vi "DAQ Engineer.vi"(0 "DAQ Name":string="USB-6343", 1 "DAQ Engr Action":T3, 5 "Channel":T2, 7 "Trigger":T1, 9 "Value":dbl, 11 "error in (no error)":errorcluster) -> (4 "device":tag, 14 "Connected":bool, 15 "error out":errorcluster)   [LabVIEW 2015]
uses:
  DAQ Engineer.ctl
  NI DAQs/NI-DAQ6343/Digital Channels.ctl
  NI DAQs/NI-DAQ6343/PFI Channels.ctl
  <vilib>/DAQmx/write.llb/DAQmx Write (Digital Wfm 1Chan NSamp).vi
  <vilib>/DAQmx/write.llb/DAQmx Write (Digital U32 1Chan 1Samp).vi
  <vilib>/Waveform/DWDTOps.llb/DWDT Boolean Array to Digital.vi
  <vilib>/DAQmx/create/channels.llb/DAQmx Create Channel (DO-Digital Output).vi
  <vilib>/DAQmx/configure/timing.llb/DAQmx Timing (Sample Clock).vi
  <vilib>/DAQmx/configure/trigger.llb/DAQmx Start Trigger (Digital Edge).vi
  <vilib>/Waveform/DWDTOps.llb/DWDT Uncompress Digital.vi
  <vilib>/DAQmx/miscellaneous.llb/DAQmx Fill In Error Info.vi
  <vilib>/DAQmx/create/channels.llb/DAQmx Create Channel (DI-Digital Input).vi
panel:
  out "Digital Waveform Graph":digitalwaveform(graph)
  out "ch":string
  out "trigger":string
  # "need three pulses for\nthe instrument to register"
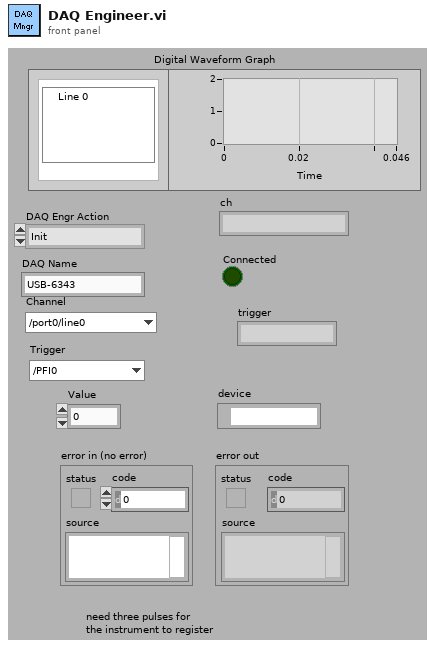
[diagram p1: front panel]
types:
  T1 = typedef "PFI Channels.ctl" = enum16{"/PFI0", "/PFI1", "/PFI2", "/PFI3", "/PFI4", "/PFI5", "/PFI6", "/PFI7", "/PFI8", "/PFI9", "/PFI10", "/PFI11", "/PFI12", "/PFI13", "/PFI14", "/PFI15"}
  T2 = typedef "Digital Channels.ctl" = enum16{"/port0/line0", "/port0/line1", "/port0/line2", "/port0/line3", "/port0/line4", "/port0/line5", "/port0/line6", "/port0/line7", "/port0/line8", "/port0/line9", "/port0/line10", "/port0/line11", "/port0/line12", "/port0/line13", "/port0/line14", "/port0/line15", "/port0/line16", "/port0/line17", "/port0/line18", "/port0/line19", "/port0/line20", "/port0/line21", "/port0/line22", "/port0/line23", "/port0/line24", "/port0/line25", "/port0/line26", "/port0/line27", "/port0/line28", "/port0/line29", "/port0/line30", "/port0/line31"}
  T3 = typedef "DAQ Engineer.ctl" = enum16{"Init", "All Digital Out", "All Digital Input", "DigitalOutOnTrigger", "Close"}
  T4 = cluster{"negative limit switch":bool, "positive limit switch":bool, "home switch":bool, "position marker":bool, "device enable":bool, "quick stop":bool, "general purpose J":bool, "general purpose I":bool, "general purpose H":bool, "general purpose G":bool, "general purpose F":bool, "general purpose E":bool, "general purpose D":bool, "general purpose C":bool, "general purpose B":bool, "general purpose A":bool}
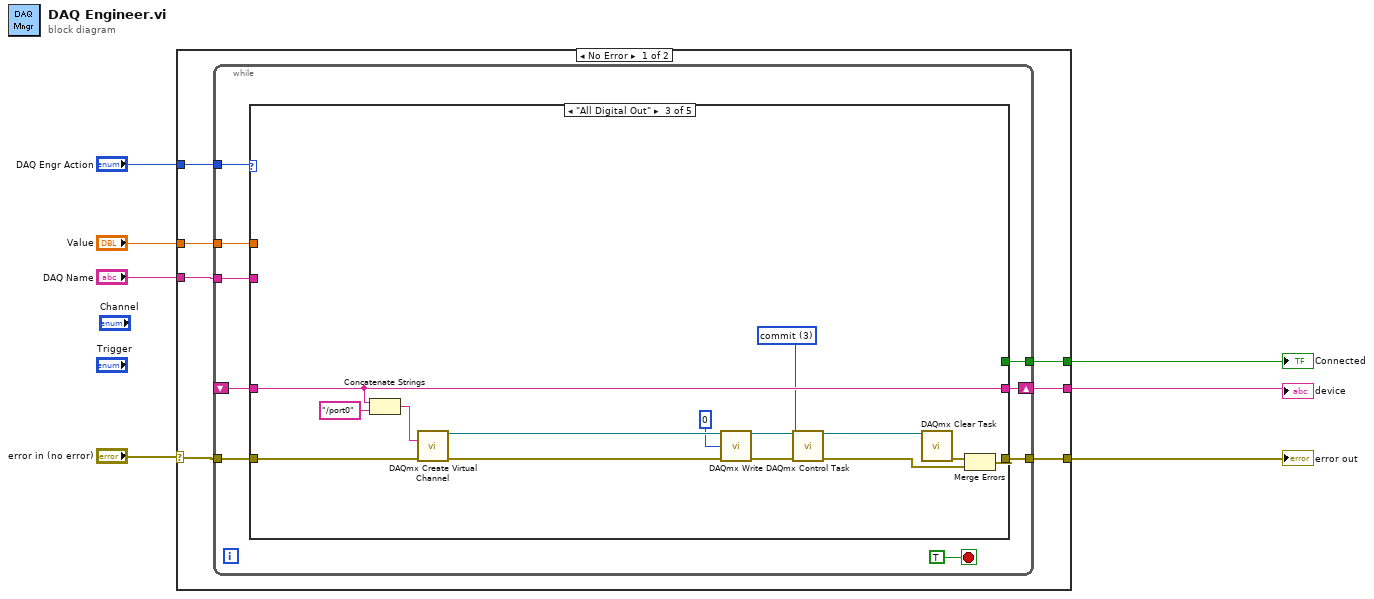
[diagram p0: block diagram]
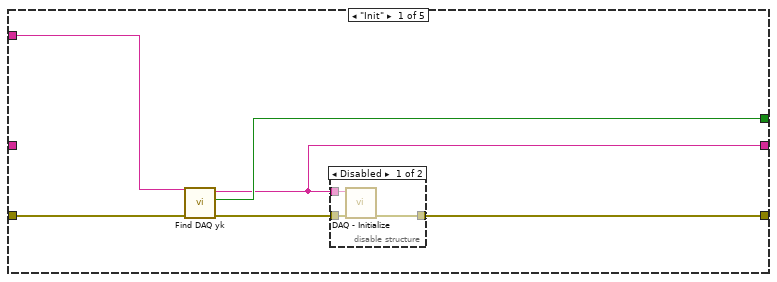
[diagram p2: hidden frame]
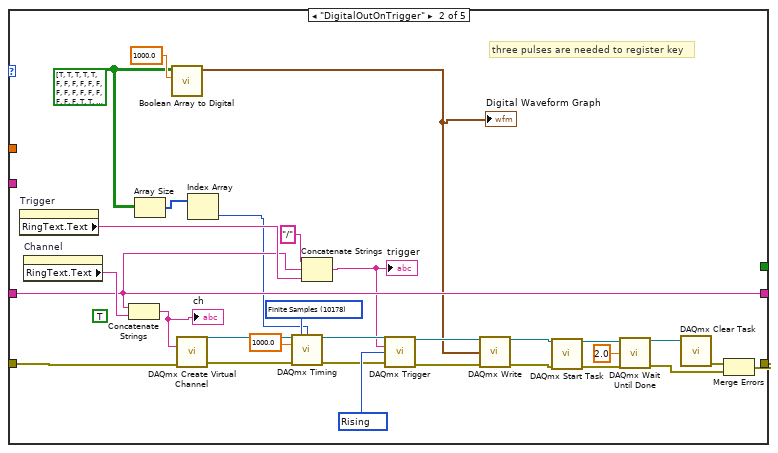
[diagram p4: hidden frame]
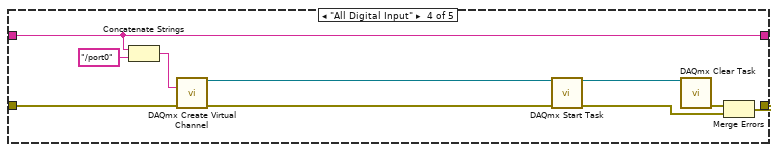
[diagram p5: hidden frame]
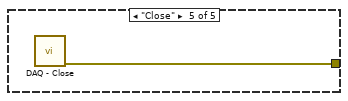
[diagram p6: hidden frame]
diagram:
  n1 = case shown="No Error" "error in (no error)" {
    selector: "error in (no error)" -> [w14 w88]
    tunnel: [w12 w88] -> w6
    tunnel: "DAQ Name" -> [w13 _]
    tunnel: "DAQ Engr Action" -> [w11 _]
    tunnel: [w10 _] -> w3
    tunnel: [w9 _] -> w2
    tunnel: "Value" -> [w8 _]
    frame No Error {
      n2 = while {
        tunnel: w14 -> [w21]
        tunnel: w13 -> [w20]
        tunnel: [w19] -> w12
        tunnel: w11 -> [w22]
        tunnel: [w18] -> w10
        tunnel: w8 -> [w16]
        shift-right: [w17] -> w9
        shift-left: _ -> [w15]
        stop <- TRUE stop-if-true
        n3 = case shown="\"All Digital Out\"" w22 {
          tunnel: w21 -> [w28 w40 w71 w83 _]
          tunnel: w20 -> [w27 _ _ _ _]
          tunnel: [w26 w51 w74 w84 w87] -> w19
          tunnel: [w25 _ _ _ _] -> w18
          tunnel: [w24 w52 w75 w85 _] -> w17
          tunnel: w16 -> [_ _ _ _ _]
          tunnel: w15 -> [_ w52 w75 w85 _]
          frame "Init" {
            n4 = call "Find DAQ yk.vi"("error in"=w28, "DAQ Name"=w27) -> ("error out"=w29:errorcluster, "Device Found"=w25:bool, "device"=w24:tag)  [unwired: 5 in, 2 out]
            n5 = disable-structure shown="Disabled" {
              disable-tunnel: w29 -> [w32 _]
              disable-tunnel: [w31 _] -> w26
              disable-tunnel: w24 -> [w30 _]
              frame Disabled {
                n6 = call "DAQ - Initialize.vi"("error in (no error)"=w32, "DAQ"=w30) -> ("error out"=w31:errorcluster)  [unwired: 9 in]
              }
              frame Enabled {
              }
            }
          }
          frame "DigitalOutOnTrigger" {
            w34 = bool[][] [[TRUE], [TRUE], [TRUE], [TRUE], [TRUE], [FALSE], [FALSE], [FALSE], [FALSE], [FALSE], [FALSE], [FALSE], [FALSE], [FALSE], [FALSE], [FALSE], [FALSE], [FALSE], [FALSE], [FALSE], [TRUE], [TRUE], [TRUE], [TRUE], [TRUE], [FALSE], [FALSE], [FALSE], [FALSE], [FALSE], [FALSE], [FALSE], [FALSE], [FALSE], [FALSE], [FALSE], [FALSE], [FALSE], [FALSE], [FALSE], [TRUE], [TRUE], [TRUE], [TRUE], [TRUE], [FALSE]] ("transposed array")
            w58 = 10178 items=["Finite Samples"=10178, "Continuous Samples"=10123, "Hardware Timed Single Point"=12522] ("sample mode")
            w60 = 10280 items=["Rising"=10280, "Falling"=10171] ("edge")
            (unwired) TRUE ("auto cleanup")
            # "three pulses are needed to register key"
            n7 = property on="Trigger" class="Enum (strict)"() -> ("RingText.Text"=w61:string)  [unwired: 2 in, 2 out]
            n8 = property on="Channel" class="Enum (strict)"() -> ("RingText.Text"=w62:string)  [unwired: 2 in, 2 out]
            n9 = Concatenate Strings(w52, w62) -> (w39:string)
            "ch" <- w39
            n10 = Array Size(array=w34) -> (size(s)=w38:i32[])
            n11 = call-poly <vilib>:"Boolean Array to Digital.vi"("sample rate"=1000.0, "boolean array"=w34) -> ("digital waveform"=w35:digitalwaveform)  [unwired: 8 in, 1 out]
            "Digital Waveform Graph" <- w35
            n12 = call-poly <vilib>:"DAQmx Create Virtual Channel.vi"("lines"=w39, "error in"=w40) -> ("task out"=w55:refnum<k21>, "error out"=w56:errorcluster)  [unwired: 12 in]
            n13 = Index Array(array=w38) -> (element=w37:i32)  [unwired: 1 in]
            n14 = call-poly <vilib>:"DAQmx Timing.vi"("task/channels in"=w55, "sample mode"=w58, "samples per channel"=w37, "rate"=1000.0, "error in"=w56) -> ("task out"=w54:refnum<k21>, "error out"=w53:errorcluster)  [unwired: 9 in]
            n15 = Concatenate Strings("/" ("Ring Text.Text"), w52, w61) -> (w33:string)
            "trigger" <- w33
            n16 = call-poly <vilib>:"DAQmx Trigger.vi"("task/channels in"=w54, "source"=w33, "edge"=w60, "error in"=w53) -> ("task out"=w49:refnum<k21>, "error out"=w50:errorcluster)  [unwired: 10 in]
            n17 = call-poly <vilib>:"DAQmx Write.vi"("task/channels in"=w49, "data"=w35, "error in"=w50) -> ("task out"=w47:refnum<k21>, "error out"=w48:errorcluster)  [unwired: 10 in, 1 out]
            n18 = call <vilib>:"DAQmx Start Task.vi"("task/channels in"=w47, "error in"=w48) -> ("task out"=w46:refnum<k21>, "error out"=w44:errorcluster)  [unwired: 12 in]
            n19 = call <vilib>:"DAQmx Wait Until Done.vi"("task/channels in"=w46, "timeout (sec)"=2.0, "error in"=w44) -> ("task out"=w45:refnum<k21>, "error out"=w43:errorcluster)  [unwired: 11 in]
            n20 = call <vilib>:"DAQmx Clear Task.vi"("task in"=w45) -> ("error out"=w59:errorcluster)  [unwired: 14 in]
            n21 = Merge Errors(w59, w43) -> (w51:errorcluster)
          }
          frame "All Digital Out" {
            w63 = 3 items=["verify"=2, "reserve"=4, "commit"=3, "unreserve"=5, "abort"=6] ("action")
            n22 = Concatenate Strings(w75, "/port0" ("string")) -> (w70:string)
            n23 = call-poly <vilib>:"DAQmx Create Virtual Channel.vi"("lines"=w70, "error in"=w71) -> ("task out"=w67:refnum<k21>, "error out"=w68:errorcluster)  [unwired: 12 in]
            n24 = call-poly <vilib>:"DAQmx Write.vi"("task/channels in"=w67, "data"=u32 0, "error in"=w68) -> ("task out"=w72:refnum<k21>, "error out"=w73:errorcluster)  [unwired: 10 in, 1 out]
            n25 = call <vilib>:"DAQmx Control Task.vi"("task/channels in"=w72, "action"=w63, "error in"=w73) -> ("task out"=w65:refnum<k21>, "error out"=w64:errorcluster)  [unwired: 11 in]
            n26 = call <vilib>:"DAQmx Clear Task.vi"("task in"=w65) -> ("error out"=w76:errorcluster)  [unwired: 14 in]
            n27 = Merge Errors(w76, w64) -> (w74:errorcluster)
          }
          frame "All Digital Input" {
            n28 = Concatenate Strings(w85, "/port0" ("string")) -> (w82:string)
            n29 = call-poly <vilib>:"DAQmx Create Virtual Channel.vi"("lines"=w82, "error in"=w83) -> ("task out"=w80:refnum<k21>, "error out"=w79:errorcluster)  [unwired: 12 in]
            n30 = call <vilib>:"DAQmx Start Task.vi"("task/channels in"=w80, "error in"=w79) -> ("task out"=w78:refnum<k21>, "error out"=w77:errorcluster)  [unwired: 12 in]
            n31 = call <vilib>:"DAQmx Clear Task.vi"("task in"=w78) -> ("error out"=w86:errorcluster)  [unwired: 14 in]
            n32 = Merge Errors(w86, w77) -> (w84:errorcluster)
          }
          frame "Close" {
            n33 = call "DAQ - Close.vi"() -> ("error out"=w87:errorcluster)  [unwired: 11 in]
          }
        }
      }
    }
    frame Error {
      (unwired) T4 {"negative limit switch"=FALSE, "positive limit switch"=FALSE, "home switch"=FALSE, "position marker"=FALSE, "device enable"=FALSE, "quick stop"=FALSE, "general purpose J"=FALSE, "general purpose I"=FALSE, "general purpose H"=FALSE, "general purpose G"=FALSE, "general purpose F"=FALSE, "general purpose E"=FALSE, "general purpose D"=FALSE, "general purpose C"=FALSE, "general purpose B"=FALSE, "general purpose A"=FALSE} ("digital inputs")
    }
  }
  "error out" <- w6
  "Connected" <- w3
  "device" <- w2
